vi "0-360_Degree_Converter.vi"(11 "Yaw in":dbl) -> (3 "Yaw out":dbl)   [LabVIEW 2017]
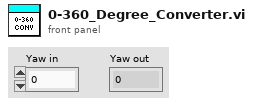
[diagram p1: front panel]
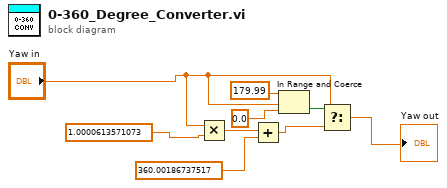
[diagram p0: block diagram]
diagram:
  n1 = Multiply(x="Yaw in", y=1.0000613571073) -> (x*y=w2:dbl)
  n2 = Add(x=w2, y=360.00186737517) -> (x+y=w4:dbl)
  n3 = In Range and Coerce(upper limit=179.99, x="Yaw in", lower limit=0.0) -> (In Range?=w5:bool)  [unwired: 1 out]
  n4 = Select(t="Yaw in", s=w5, f=w4) -> (s? t:f=→"Yaw out":dbl)
